vi "AOM waveform.vi"(7 "z stack 往复采样信息":cluster{"Fs":dbl, "#s":dbl}, 9 "AOM Blind percent (%)":dbl, 10 "AOM start blind percent (%)":dbl, 11 "Bi-Lateral Galvo xy scan frequency (Hz)":i16) -> (2 "数值":i32, 3 "Waveform":waveform(dbl))   [LabVIEW 2018]
uses:
  <vilib>/measure/NI_MABase.lvlib
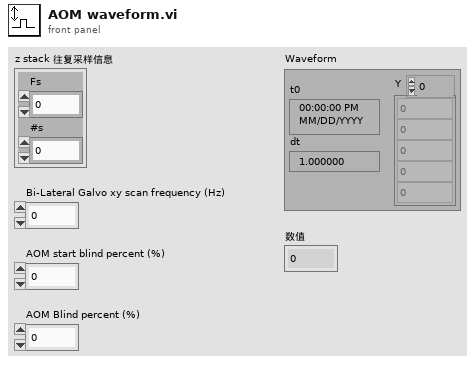
[diagram p1: front panel]
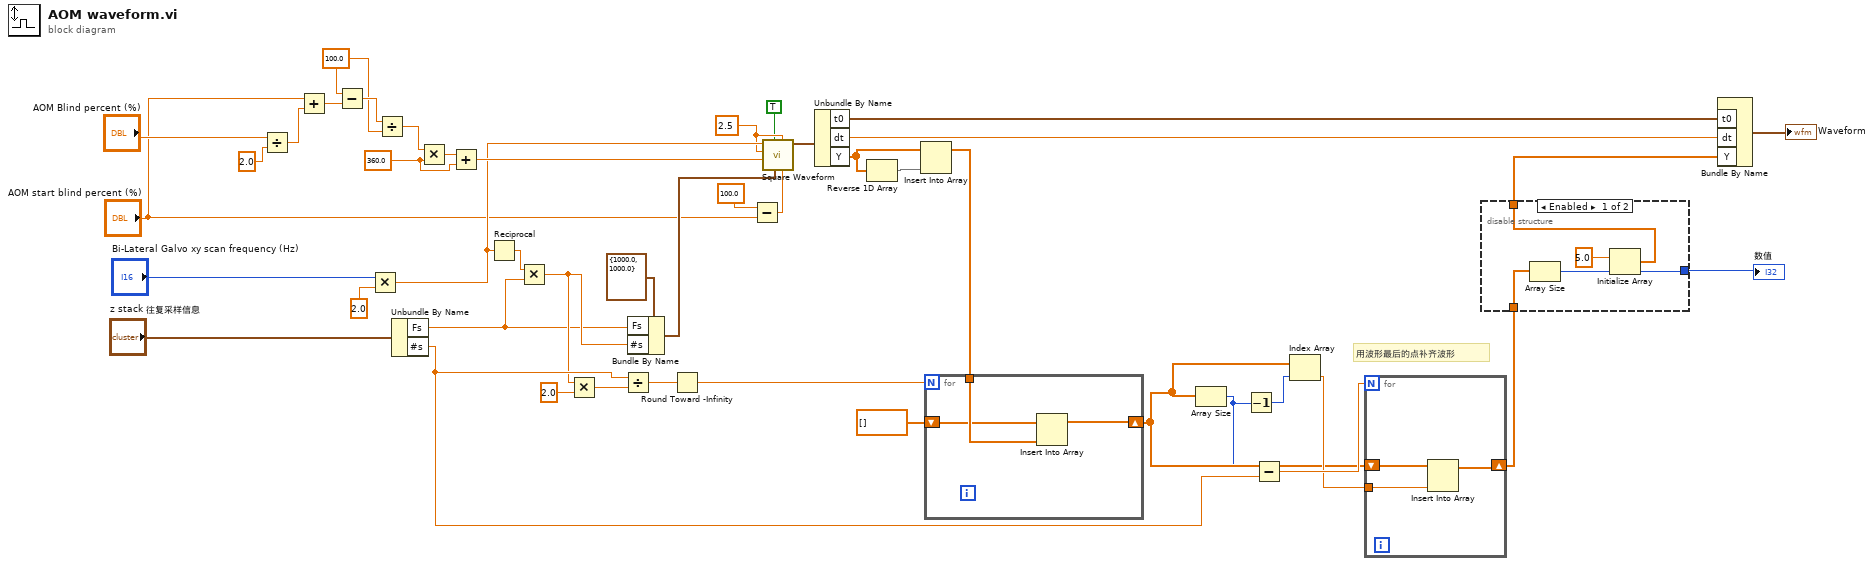
[diagram p0: block diagram]
diagram:
  w40 = 360.0 ("y")
  w36 = 100.0 ("y")
  w8 = 2.5 ("y")
  # "用波形最后的点补齐波形"
  n1 = Divide(x="AOM Blind percent (%)", y=2.0) -> (x/y=w34:dbl)
  n2 = Add(x="AOM start blind percent (%)", y=w34) -> (x+y=w35:dbl)
  n3 = Subtract(x=w36, y=w35) -> (x-y=w37:dbl)
  n4 = Multiply(x="Bi-Lateral Galvo xy scan frequency (Hz)", y=2.0) -> (x*y=w14:dbl)
  n5 = Divide(x=w37, y=w36) -> (x/y=w38:dbl)
  n6 = Unbundle By Name("z stack 往复采样信息") -> ("Fs"=w16:dbl, "#s"=w45:dbl)
  n7 = Multiply(x=w38, y=w40) -> (x*y=w39:dbl)
  n8 = Add(x=w39, y=w40) -> (x+y=w41:dbl)
  n9 = Reciprocal(x=w14) -> (1/x=w15:dbl)
  n10 = Multiply(x=w15, y=w16) -> (x*y=w22:dbl)
  n11 = Multiply(x=w22, y=2.0) -> (x*y=w24:dbl)
  n12 = Divide(x=w45, y=w24) -> (x/y=w25:dbl)
  n13 = Bundle By Name(cluster=cluster{"Fs":dbl, "#s":dbl} {"Fs"=1000.0, "#s"=1000.0} ("sampling info"), "Fs"=w16, "#s"=w22) -> (w11:cluster{"Fs":dbl, "#s":dbl})
  n14 = Round Toward -Infinity(1:w25) -> (0:w26:dbl)
  n15 = Subtract(x=100.0, y="AOM start blind percent (%)") -> (x-y=w13:dbl)
  n16 = call <vilib>:"Square Waveform.vi"("duty cycle (%)"=w13, "offset"=w8, "sampling info"=w11, "reset signal"=TRUE, "phase"=w41, "amplitude"=w8, "frequency"=w14) -> ("signal out"=w17:waveform(dbl))  [unwired: 3 in, 1 out]
  n17 = Unbundle By Name(w17) -> ("t0"=w44:timestamp, "dt"=w43:dbl, "Y"=w18:dbl[])
  n18 = Reverse 1D Array(array=w18) -> (reversed array=w19:dbl[])
  n19 = Insert Into Array(array=w18, new element=w19) -> (w21:dbl[])  [unwired: 1 in]
  n20 = for {
    N: w26 -> [_]
    shift-right: [w46] -> w29
    shift-left: dbl[] [] -> [w47]
    tunnel: w21 -> [w48]
    n21 = Insert Into Array(array=w47, new element=w48) -> (w46:dbl[])  [unwired: 1 in]
  }
  n22 = Array Size(array=w29) -> (size(s)=w27:i32)
  n23 = Decrement(x=w27) -> (x-1=w28:i32)
  n24 = Subtract(x=w27, y=w45) -> (x-y=w31:dbl)
  n25 = Index Array(array=w29, index=w28) -> (element=w30:dbl)
  n26 = for {
    N: w31 -> [_]
    shift-right: [w49] -> w42
    shift-left: w29 -> [w51]
    tunnel: w30 -> [w50]
    n27 = Insert Into Array(array=w51, new element=w50) -> (w49:dbl[])  [unwired: 1 in]
  }
  n28 = disable-structure shown="Enabled" {
    disable-tunnel: w42 -> [w53 w56]
    disable-tunnel: [w55 _] -> w2
    disable-tunnel: [w52 w56] -> w1
    frame Enabled {
      n29 = Array Size(array=w53) -> (size(s)=w55:i32)
      n30 = Initialize Array(5.0 ("element"), w55) -> (w52:dbl[])
    }
    frame Disabled {
    }
  }
  "数值" <- w2
  n31 = Bundle By Name("t0"=w44, "dt"=w43, "Y"=w1) -> (→"Waveform":waveform(dbl))  [unwired: 1 in]
